vi "Create_Keithley_Scan_Files.vi"(8 "error in (no error)":errorcluster, 11 "base path":path) -> (0 "error out":errorcluster, 1 "New Folder Created?":bool, 2 "Ref Num Array":refnum<file>[](array[refnum]), 3 "Save Files Array":path[](array[path]), 4 "Scan Number":i32)   [LabVIEW 2018]
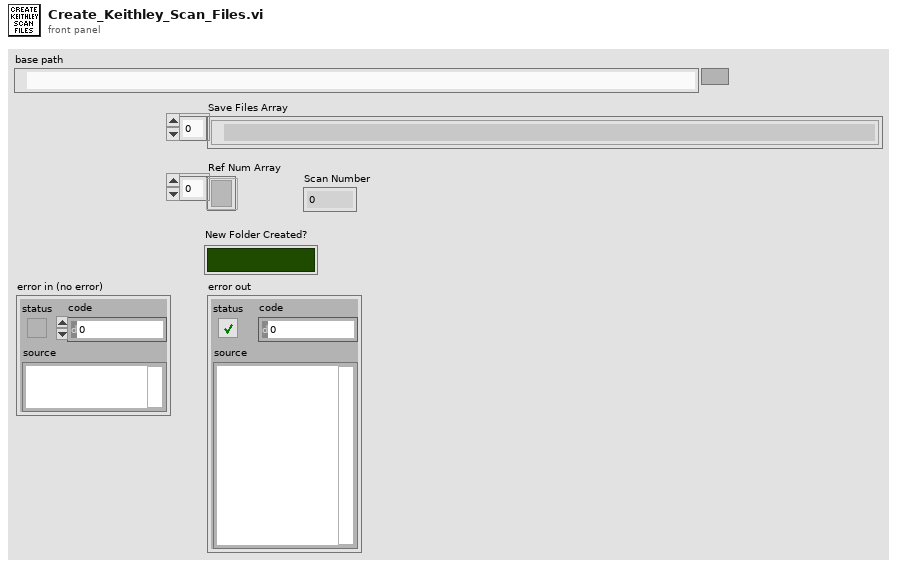
[diagram p1: front panel]
types:
  T1 = enum16{"open", "replace", "create", "open or create", "replace or create", "replace or create with confirmation"}
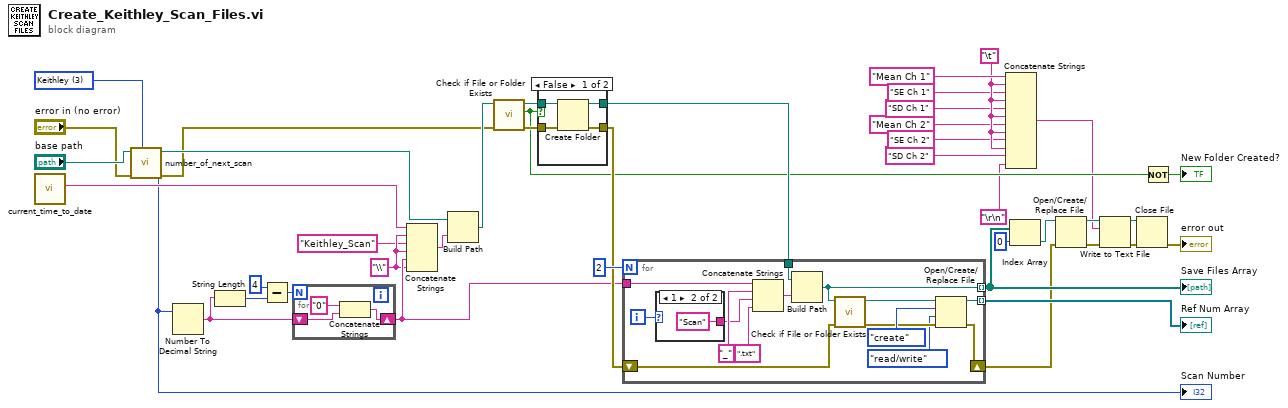
[diagram p0: block diagram]
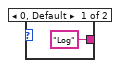
[diagram p3: hidden frame]
diagram:
  w7 = "\t"
  w9 = u16 3 items=["Energy / Time", "Motor", "TDC", "Keithley", "Pressure Scan"] ("Scan Type")
  w28 = "\\" ("string")
  n1 = call "current_time_to_date.vi"() -> ("yyyy-mm-dd"=w37:string)  [unwired: 10 in, 1 out]
  n2 = call "number_of_next_scan.vi"("Scan Type"=w9, "error in (no error)"="error in (no error)", "base path"="base path") -> ("error out"=w22:errorcluster, "scan nr"=w11:i32, "path out"=w24:path)  [unwired: 6 in]
  "Scan Number" <- w11
  n3 = Number To Decimal String(number=w11) -> (decimal integer string=w39:string)  [unwired: 1 in]
  n4 = String Length(string=w39) -> (length=w42:i32)
  n5 = Subtract(x=4, y=w42) -> (x-y=w40:i32)
  n6 = for {
    N: w40 -> [_]
    shift-right: [w43] -> w29
    shift-left: w39 -> [w44]
    n7 = Concatenate Strings("0", w44) -> (w43:string)
  }
  n8 = Concatenate Strings(w37, w28, "Keithley_Scan" ("string"), w28, w29, w28) -> (w32:string)
  n9 = Build Path(base path=w24, name or relative path=w32) -> (appended path=w36:path)
  n10 = call <vilib>:"Check if File or Folder Exists.vi"("error in (no error)"=w22, "path"=w36) -> ("error out"=w33:errorcluster, "file or folder exists?"=w27:bool, "dup path"=w35:path)  [unwired: 7 in]
  n11 = case shown="False" w27 {
    tunnel: w35 -> [w49 w51]
    tunnel: [w48 w51] -> w34
    tunnel: w33 -> [w47 w50]
    tunnel: [w46 w50] -> w31
    frame False {
      n12 = Create Folder(path (use dialog)=w49, error in=w47) -> (created path=w48:path, error out=w46:errorcluster)  [unwired: 1 in, 1 out]
    }
    frame True {
    }
  }
  n13 = for {
    N: 2 -> [_]
    tunnel: w29 -> [w65]
    tunnel: w34 -> [w64]
    tunnel: [w59] -> w21 mode=indexing
    shift-right: [w54] -> w14
    shift-left: w31 -> [w55]
    tunnel: [w52] -> w30 mode=indexing
    i -> [w61]
    n14 = case shown="1" w61 {
      tunnel: ["Log" ("string") "Scan" ("string")] -> w60
      frame 0, Default {
      }
      frame 1 {
      }
    }
    n15 = Concatenate Strings(w65, "_" ("string"), w60, ".txt" ("string")) -> (w66:string)
    n16 = Build Path(base path=w64, name or relative path=w66) -> (appended path=w59:path)
    n17 = call <vilib>:"Check if File or Folder Exists.vi"("error in (no error)"=w55, "path"=w59) -> ("error out"=w56:errorcluster, "dup path"=w58:path)  [unwired: 7 in, 1 out]
    n18 = Open/Create/Replace File(file path (use dialog)=w58, error in=w56, operation (0:open)=T1."create", access (0:read/write)=enum16{"read/write", "read-only", "write-only"}."read/write") -> (refnum out=w52:refnum<file>, error out=w54:errorcluster)  [unwired: 2 in, 1 out]
  }
  "Save Files Array" <- w21
  "Ref Num Array" <- w30
  n19 = Concatenate Strings("Mean Ch 1" ("string"), w7, "SE Ch 1" ("string"), w7, "SD Ch 1" ("string"), w7, "Mean Ch 2" ("string"), w7, "SE Ch 2" ("string"), w7, "SD Ch 2" ("string"), "\r\n") -> (w12:string)
  n20 = Index Array(array=w21, index=0) -> (element=w19:path)
  n21 = Open/Create/Replace File(file path (use dialog)=w19, error in=w14) -> (refnum out=w17:refnum<file>, error out=w18:errorcluster)  [unwired: 4 in, 1 out]
  n22 = Write to Text File(file (use dialog)=w17, text=w12, error in=w18) -> (refnum out=w16:refnum<file>, error out=w15:errorcluster)  [unwired: 1 in, 1 out]
  n23 = Close File(refnum=w16, error in=w15) -> (error out=→"error out":errorcluster)  [unwired: 1 out]
  n24 = Not(x=w27) -> (.not. x?=→"New Folder Created?":bool)
